vi "Get Scroll.vi"(8 "error in (no error)":errorcluster, 11 "2DArrayManager in":refnum<class "2DArrayManager.lvclass">) -> (0 "error out":errorcluster, 2 "Scroll":T1, 3 "2DArrayManager out":refnum<class "2DArrayManager.lvclass">)   [LabVIEW 2020, in "OOPanel.lvlib" / "2DArrayManager.lvclass"]
uses:
  2DArrayManager.lvclass
  2D Position.ctl
  OOPanel.lvlib
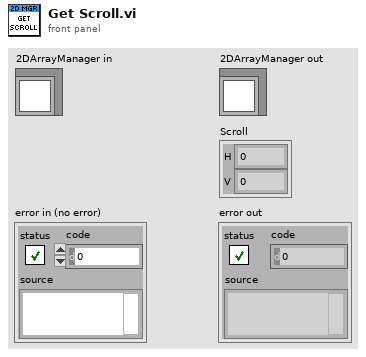
[diagram p1: front panel]
types:
  T1 = typedef "OOPanel.lvlib/2D Position.ctl" = cluster{"H":i32, "V":i32}
  T2 = typedef "OOPanel.lvlib/2DArrayManager.lvclass/State.ctl" = cluster{"Scroll":T1, "Scroll Max":T1, "Top-Left Index":T3, "H Scroll Sync":refnum<user-event>, "V Scroll Sync":refnum<user-event>, "Sync":bool, "H Scroll Vis":bool, "V Scroll Vis":bool, "Blank Pool":refnum<queue>}
  T3 = typedef "OOPanel.lvlib/2D Index.ctl" = cluster{"Row":i32, "Col":i32}
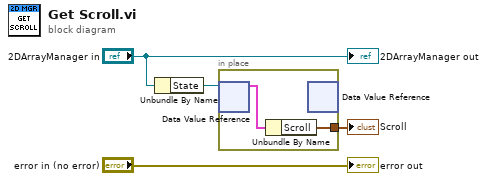
[diagram p0: block diagram]
diagram:
  n1 = Unbundle By Name("2DArrayManager in") -> ("State"=w3:refnum<data-value>)
  n2 = in-place {
    in-place-border: [w5] -> w1
    n3 = in-place-dvr #1(w3) -> (w6:T2)  [unwired: 1 out]
    n4 = Unbundle By Name(w6) -> ("Scroll"=w5:T1)
    n5 = in-place-dvr #1() -> ()  [unwired: 1 in, 2 out]
  }
  "Scroll" <- w1
  "error out" <- "error in (no error)"
  "2DArrayManager out" <- "2DArrayManager in"
